vi "Gyroscope Reset.vi"(8 "error in (no error)":errorcluster, 11 "Gyroscope in":refnum<class "IMU.lvclass">) -> (0 "error out":errorcluster, 3 "Gyroscope":refnum<class "IMU.lvclass">)   [LabVIEW 2020]
uses:
  <vilib>/High Genius/HG_WSI_Tookit/Dependencies/Library/IMU/IMU.lvclass
  <vilib>/High Genius/HG_WSI_Tookit/Dependencies/Library/VMX Library.lvlib
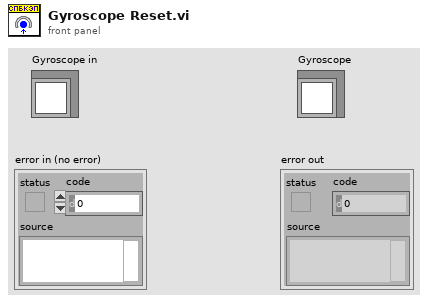
[diagram p1: front panel]
types:
  T1 = typedef "Semaphore RefNum" = refnum<k1>
  T2 = cluster{"titanenc0":i32, "titanenc1":i32, "titanenc2":i32, "titanenc3":i32, "rpm0":i16, "rpm1":i16, "rpm2":i16, "rpm3":i16, "resetenc0":bool, "resetenc1":bool, "resetenc2":bool, "resetenc3":bool}
  T3 = cluster{"data":cluster{"ai22":sgl, "ai23":sgl, "ai24":sgl, "ai25":sgl, "pulse12":i32, "pulse13":i32, "pwm14":i32, "pwm15":i32, "pwm16":dbl, "do17":bool, "do18":bool, "do19":bool, "do20":bool, "do21":bool, "di11":bool, "di9":bool, "motor0":u8, "motor1":u8, "motor2":u8, "motor3":u8, "dir00":u8, "dir01":u8, "dir02":u8, "dir03":u8, "dir10":u8, "dir11":u8, "dir12":u8, "dir13":u8, "limit0":bool, "limit1":bool, "limit2":bool, "limit3":bool, "limit4":bool, "limit5":bool, "limit6":bool, "limit7":bool, "lsb0H":u8, "lsb1H":u8, "lsb2H":u8, "lsb3H":u8, "lsb0L":u8, "lsb1L":u8, "lsb2L":u8, "lsb3L":u8, "enc0_counters":u32, "enc1_counters":u32, "enc2_counters":u32, "enc3_counters":u32, "counter10":u32, "counter8":u32, "reset_enc0":bool, "reset_enc1":bool, "reset_enc2":bool, "reset_enc3":bool, "pitch":sgl, "roll":sgl, "yaw":sgl, "zero_yaw":bool}}
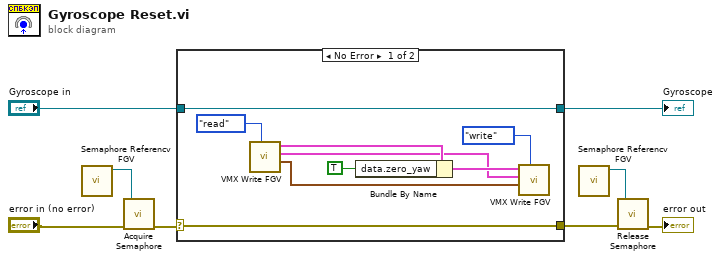
[diagram p0: block diagram]
diagram:
  n1 = call <vilib>:"Semaphore Referencv FGV.vi"() -> ("Semaphore Reference"=w1:T1)  [unwired: 11 in]
  n2 = call <vilib>:"Acquire Semaphore.vi"("error in (no error)"="error in (no error)", "semaphore"=w1) -> ("error out"=w3:errorcluster)  [unwired: 3 in, 2 out]
  n3 = case shown="No Error" w3 {
    selector: w3 -> [w16 w19]
    tunnel: [w16 w19] -> w5
    tunnel: [w17 w18] -> w7
    tunnel: "Gyroscope in" -> [w17 w18]
    frame No Error {
      n4 = call <vilib>:"VMX Write FGV.vi"("Enum"=enum16{"read", "write"}."read") -> ("Read Data3"=w9:cluster{"pwm17":i32, "pwm18":i32}, "Read Data2"=w10:T2, "Read Data"=w11:T3)  [unwired: 8 in]
      n5 = Bundle By Name(cluster=w11, "data.zero_yaw"=TRUE) -> (w14:T3)
      n6 = call <vilib>:"VMX Write FGV.vi"("Enum"=enum16{"read", "write"}."write", "Write Data3"=w9, "Write Data2"=w10, "Write Data"=w14) -> ()  [unwired: 5 in, 3 out]
    }
    frame Error {
    }
  }
  "Gyroscope" <- w7
  n7 = call <vilib>:"Semaphore Referencv FGV.vi"() -> ("Semaphore Reference"=w6:T1)  [unwired: 11 in]
  n8 = call <vilib>:"Release Semaphore.vi"("error in (no error)"=w5, "semaphore"=w6) -> ("error out"=→"error out":errorcluster)  [unwired: 4 in, 1 out]
